vi "set_scan_specification.vi"(7 "z/intensity tuples (U32: high U16 is z, low U16 is intensity)":u32[](array[numeric]), 8 "error in (no error)":errorcluster, 9 "extra waitlines array":u32[](array[numeric]), 10 "scan specification":T1, 11 "FPGA_AK101022Resonance in":refnum<class "FPGAWrapperAK101022Resonance.lvclass">) -> (0 "error out":errorcluster, 3 "FPGA_AK101022Resonance out":refnum<class "FPGAWrapperAK101022Resonance.lvclass">)   [LabVIEW 2010, in "FPGAWrapperAK101022Resonance.lvclass"]
uses:
  FPGAWrapperAK101022Resonance.lvclass
  scan_specification_cluster.ctl
  class_data.vi
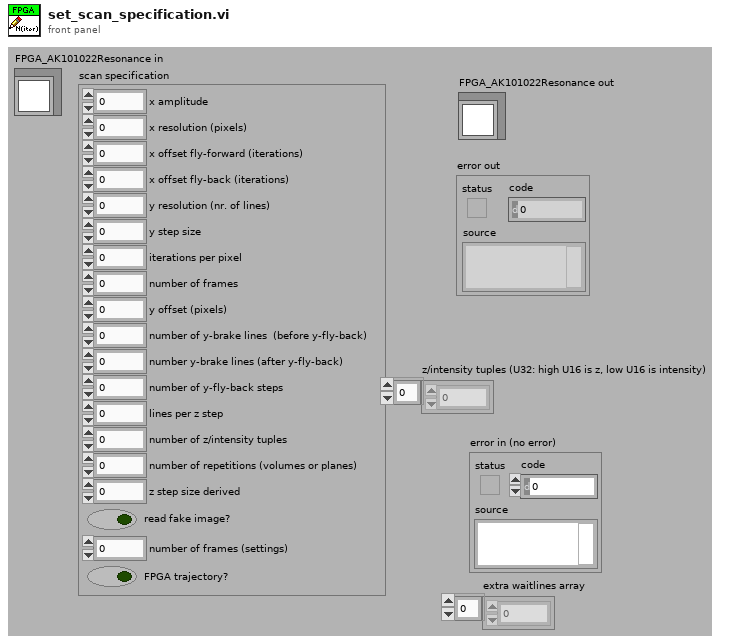
[diagram p1: front panel]
types:
  T1 = typedef "scan_specification_cluster.ctl" = cluster{"x amplitude":u16, "x resolution (pixels)":u16, "x offset fly-forward (iterations)":u16, "x offset fly-back (iterations)":u16, "y resolution (nr. of lines)":u16, "y step size":u16, "iterations per pixel":u16, "number of frames":i32, "y offset (pixels)":u16, "number of y-brake lines  (before y-fly-back)":u16, "number y-brake lines (after y-fly-back)":u16, "number of y-fly-back steps":u16, "lines per z step":u16, "number of z/intensity tuples":u16, "number of repetitions (volumes or planes)":i32, "z step size derived":u16, "read fake image?":bool, "number of frames (settings)":i32, "FPGA trajectory?":bool}
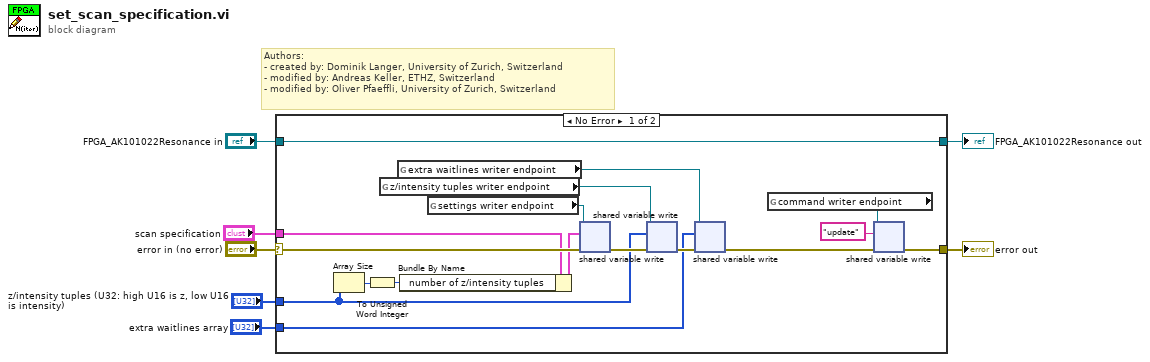
[diagram p0: block diagram]
diagram:
  # "Authors: \n- created by: Dominik Langer, University of Zurich, Switzerland\n- modified by: Andreas Keller, ETHZ, Switzerland\n- modified by: Oliver Pfaeffli, University of Zurich, Switzerland"
  n1 = case shown="No Error" "error in (no error)" {
    selector: "error in (no error)" -> [w19 w26]
    tunnel: [w23 w26] -> w5
    tunnel: [w24 w25] -> w4
    tunnel: "FPGA_AK101022Resonance in" -> [w24 w25]
    tunnel: "scan specification" -> [w16 _]
    tunnel: "z/intensity tuples (U32: high U16 is z, low U16 is intensity)" -> [w12 _]
    tunnel: "extra waitlines array" -> [w8 _]
    frame No Error {
      n2 = Array Size(array=w12) -> (size(s)=w18:i32)
      n3 = To Unsigned Word Integer(number=w18) -> (unsigned 16bit integer=w17:u16)
      n4 = global read "class_data.vi" "z/intensity tuples writer endpoint"() -> (w13:refnum<k21>)
      n5 = global read "class_data.vi" "extra waitlines writer endpoint"() -> (w9:refnum<k21>)
      n6 = Bundle By Name(cluster=w16, "number of z/intensity tuples"=w17) -> (w15:T1)
      n7 = global read "class_data.vi" "settings writer endpoint"() -> (w20:refnum<k21>)
      n8 = shared-variable-write(w20, w19, w15) -> (w14:errorcluster)  [unwired: 1 in, 2 out]
      n9 = shared-variable-write(w13, w14, w12) -> (w11:errorcluster)  [unwired: 1 in, 2 out]
      n10 = shared-variable-write(w9, w11, w8) -> (w10:errorcluster)  [unwired: 1 in, 2 out]
      n11 = global read "class_data.vi" "command writer endpoint"() -> (w22:refnum<k21>)
      n12 = shared-variable-write(w22, w10, "update" ("data in")) -> (w23:errorcluster)  [unwired: 1 in, 2 out]
    }
    frame Error {
    }
  }
  "error out" <- w5
  "FPGA_AK101022Resonance out" <- w4
